vi "TC Max and Min Benchmark.vi"() -> ()   [LabVIEW 2010]
uses:
  <vilib>/eio/EIONode/EIONode.xnode
  <vilib>/rvi/eio/nirviEIOImplementation/nirviEIOImplementation.xnode
  <vilib>/rvi/eio/common/nirviEmuClasses.ctl
  <vilib>/rvi/eio/common/nirviEmuTemplateMethod_noerrors.vi
panel:
  out "Minimum Reached":fxp<+/-,24,-2> format="%.26g"
  out "Maximum Reached":fxp<+/-,24,-2> format="%.26g"
  out "Loop Period (ticks)":u32
  out "Current TC Signal":fxp<+/-,24,-2> format="%.26g"
  # "Loop Period = ~27149454 ticks\n\n2714954 ticks * 1 s / 40,000,000 ticks = .204 s = 68 ms\n\nfor 9211, conversion time = 70ms per channel"
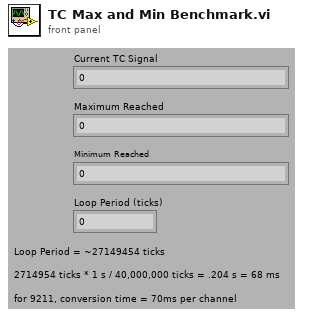
[diagram p1: front panel]
types:
  T1 = typedef "nirviEmuClasses.ctl" = enum16{"IO Read", "IO Write", "Method", "Property Read", "Property Write"}
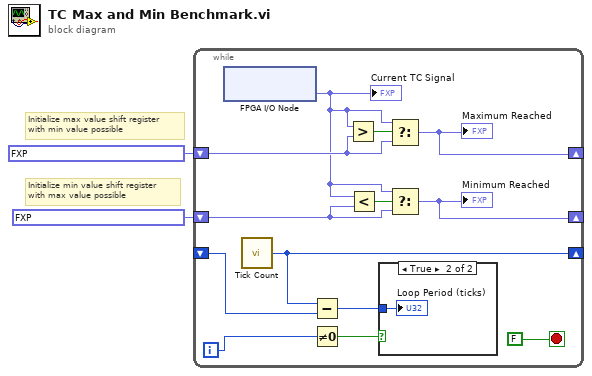
[diagram p0: block diagram]
diagram:
  # "Initialize max value shift register\nwith min value possible"
  # "Initialize min value shift register\nwith max value possible"
  n1 = while {
    shift-right: [w14] -> _
    shift-left: _ -> [w15]
    shift-right: [w7] -> _
    shift-left: fxp<+/-,24,-2> -0.125 -> [w8]
    shift-right: [w3] -> _
    shift-left: fxp<+/-,24,-2> 0.1249999850988388 -> [w4]
    i -> [w12]
    stop <- FALSE stop-if-true
    n2 = xnode "FPGA I/O Node"() -> ("Mod1/TC0"=w5:fxp<+/-,24,-2>)  [unwired: 1 in, 1 out]
    "Current TC Signal" <- w5
    n3 = call "Tick Count"() -> ("Tick Count(Ticks)"=w14:u32)
    n4 = Subtract(x=w14, y=w15) -> (x-y=w10:u32)
    n5 = Not Equal To 0?(x=w12) -> (x != 0?=w11:bool)
    n6 = Greater?(x=w5, y=w8) -> (0:w9:bool)
    n7 = Less?(x=w5, y=w4) -> (x < y?=w6:bool)
    n8 = case shown="True" w11 {
      tunnel: w10 -> [_ w16]
      frame False {
      }
      frame True {
        "Loop Period (ticks)" <- w16
      }
    }
    n9 = Select(t=w5, s=w9, f=w8) -> (s? t:f=w7:fxp<+/-,24,-2>)
    "Maximum Reached" <- w7
    n10 = Select(t=w5, s=w6, f=w4) -> (s? t:f=w3:fxp<+/-,24,-2>)
    "Minimum Reached" <- w3
  }
